vi "Additional Channels.vi"   [LabVIEW 2022 SP3]
uses:
  Controls/Post_Process.ctl
  Globals/Meas_global.vi
types:
  T1 = typedef "Analysis_info_cluster.ctl" = cluster{"Colour":u32, "Inst type":T2, "Inst name":string, "Symbol":string, "Code name":string, "Extra Info":string, "Inst Array":T3, "Extra Titles":string[], "Extra Values":string[], "U":dbl, "u^2":dbl, "u^3":dbl, "u^4":dbl, "Skew_u":dbl, "Kurt_u":dbl, "Sd Error in Mean":dbl, "% u'/U":dbl, "X":dbl, "Y":dbl, "Z":dbl, "Timescale integral Estimate":dbl, "Sd Error in Variance":dbl, "Calib File":path, "Calib Constants":dbl[], "Output Position":bool, "Stats":enum16{"None", "Basic", "Full"}, "Av Sampling Rate":dbl, "Av No of Samples":dbl, "Total Meas Time (s)":dbl, "ADAM Ch Name":string, "Max value":dbl, "Min value":dbl, "Req Sample Rate Hz":dbl, "Sync Delay Time (s)":dbl, "Ch No":i16, "Device":string, "Use Latest Calib":bool, "Port":string, "Metadata Ch Names":string[], "Metadata Ch Values":string[], "Label":string, "chState":T4}
  T2 = typedef "Inst_type.ctl" = enum16{"Raw voltage", "Raw with zero offsetting", "Propeller anemometer", "Pressure Transducer", "Pitot-static tube", "Hot wire", "Cross wire 1", "Cross wire 2", "Generic Linear", "Generic Polynomial", "Generic BackPoly", "Fast FID", "Thermocouple", "Cold wire", "Pulsed Wire", "LDA Vel", "LDA Tran time", "LDA Arr time", "Microphone"}
  T3 = typedef "Instrument_Array.ctl" = enum16{"PWA", "LDA", "Analogue"}
  T4 = typedef "channelState.ctl" = enum32{"No Selection", "Solo", "Mute"}
  T5 = typedef "Post_Process.ctl" = enum16{"Take New Data", "Post Process Raw Data File"}
  T6 = typedef "Initial Info Cluster.ctl" = cluster{"Metadata Ch Names":string[], "Metadata Ch Values":string[]}
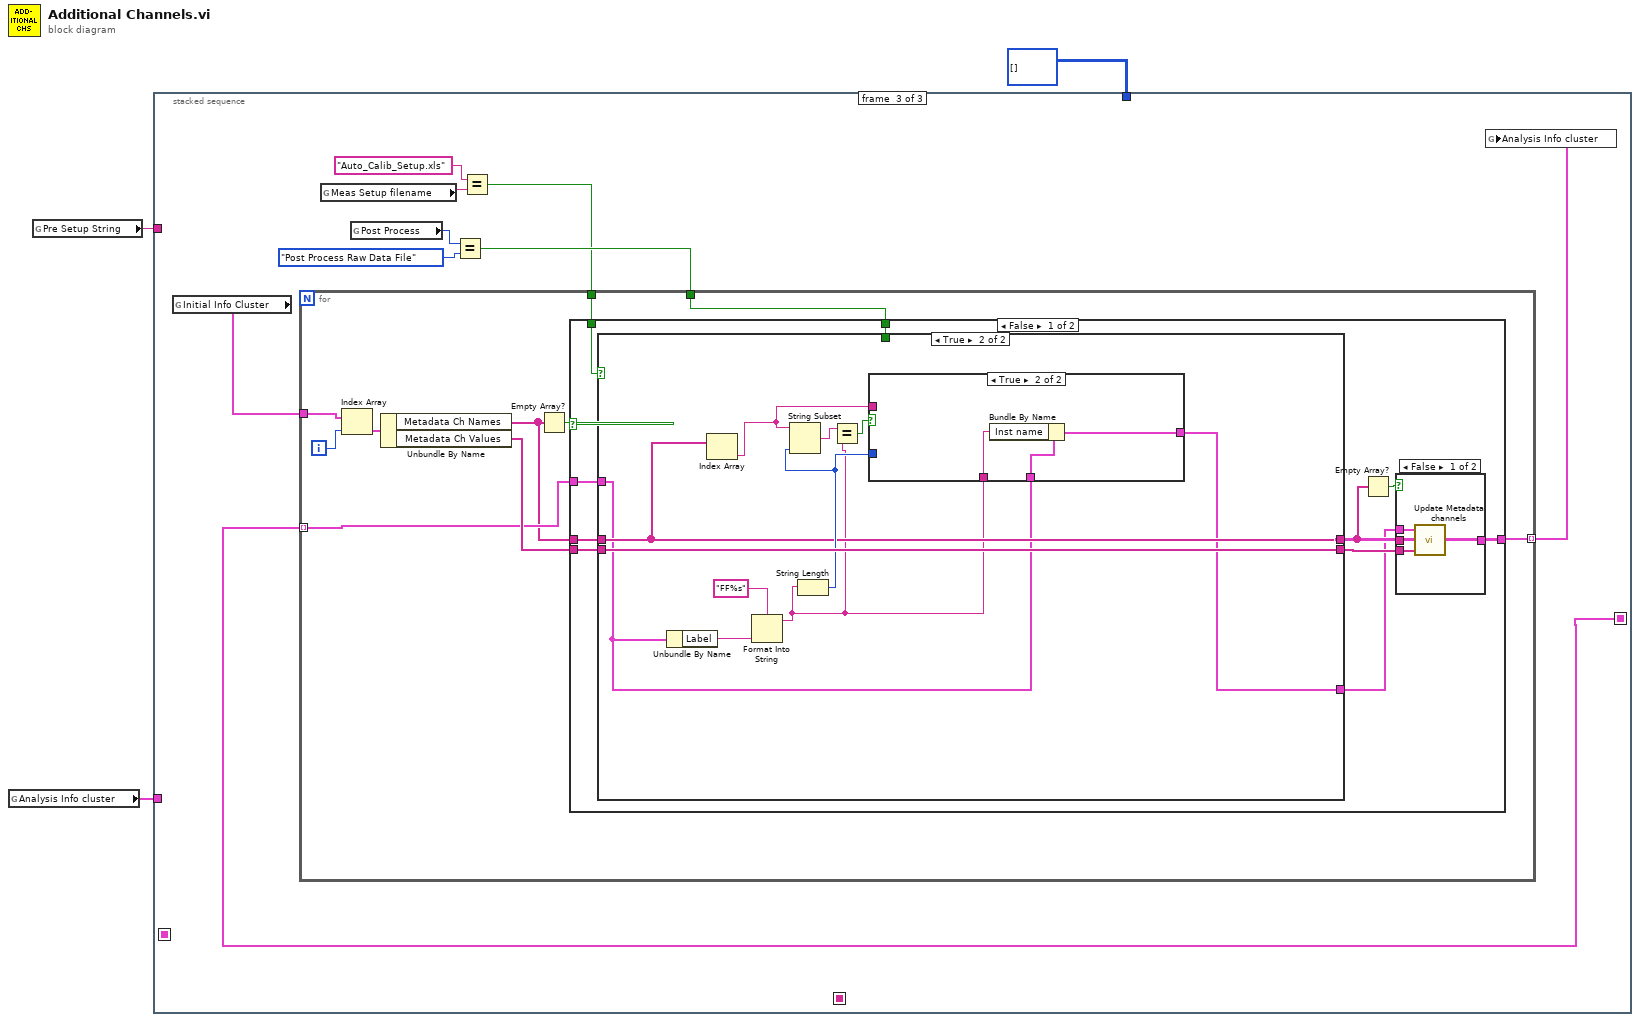
[diagram p0: block diagram]
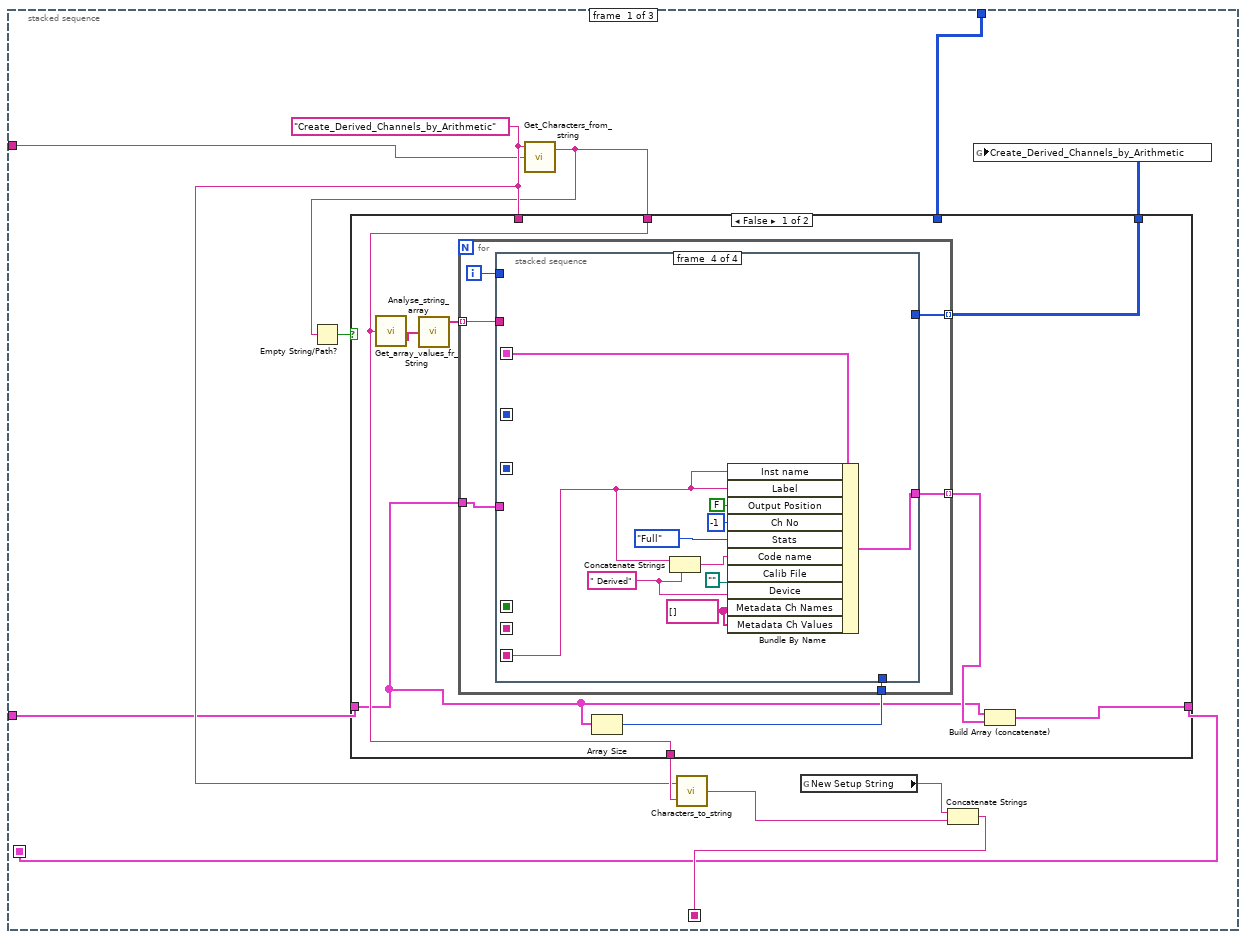
[diagram p2: hidden frame]
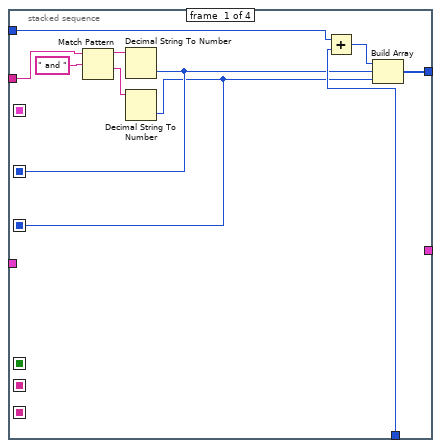
[diagram p3: hidden frame]
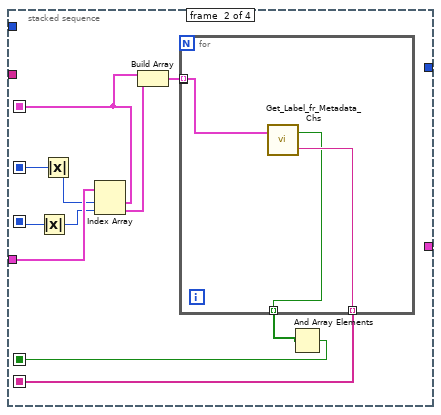
[diagram p4: hidden frame]
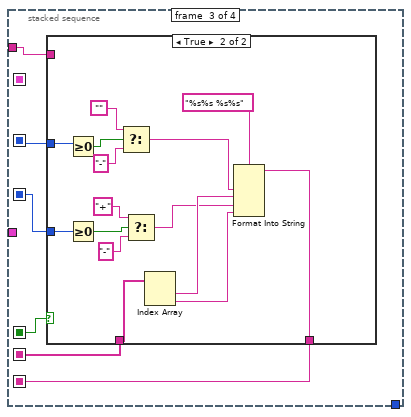
[diagram p5: hidden frame]
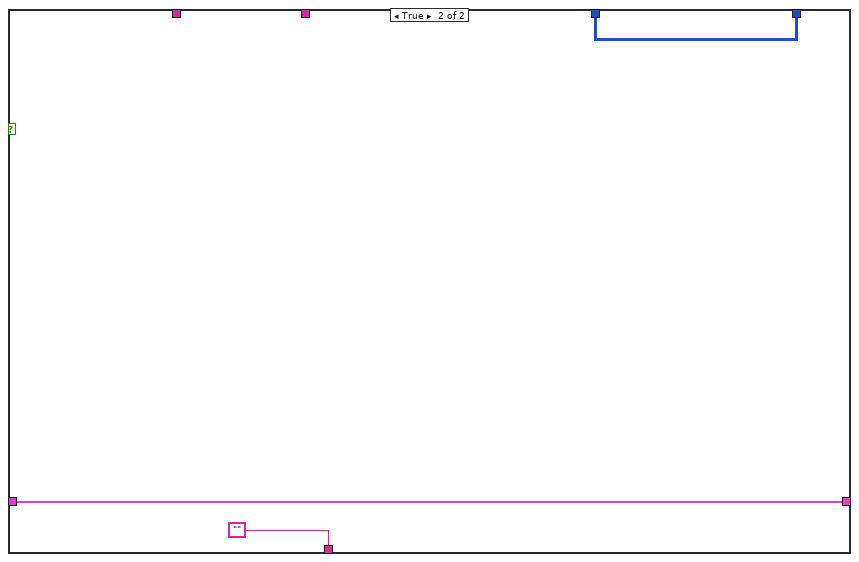
[diagram p7: hidden frame]
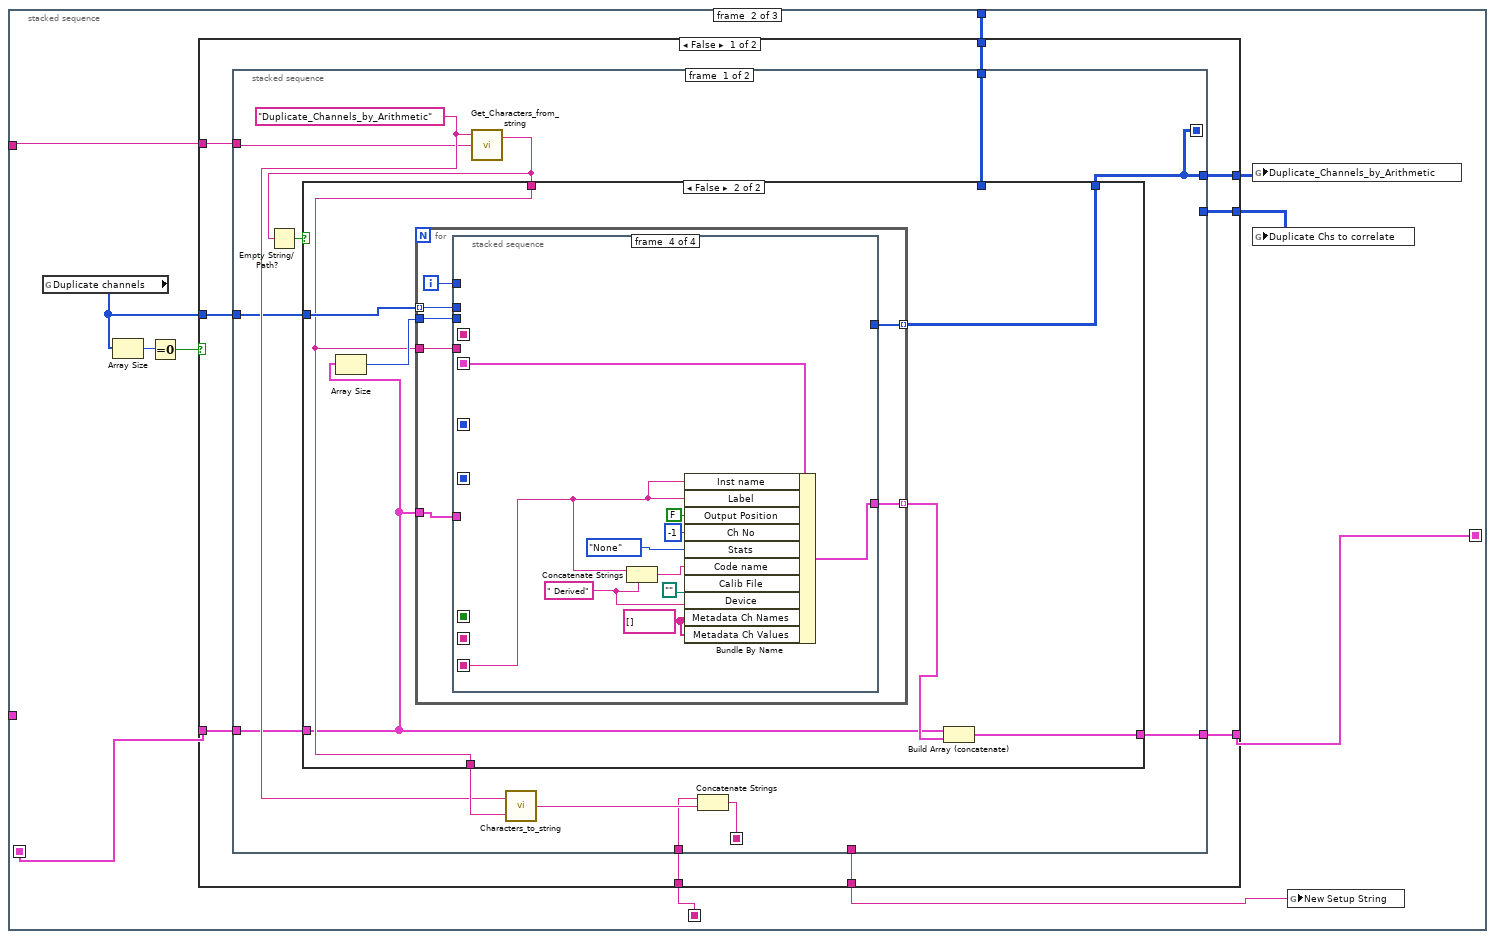
[diagram p8: hidden frame]
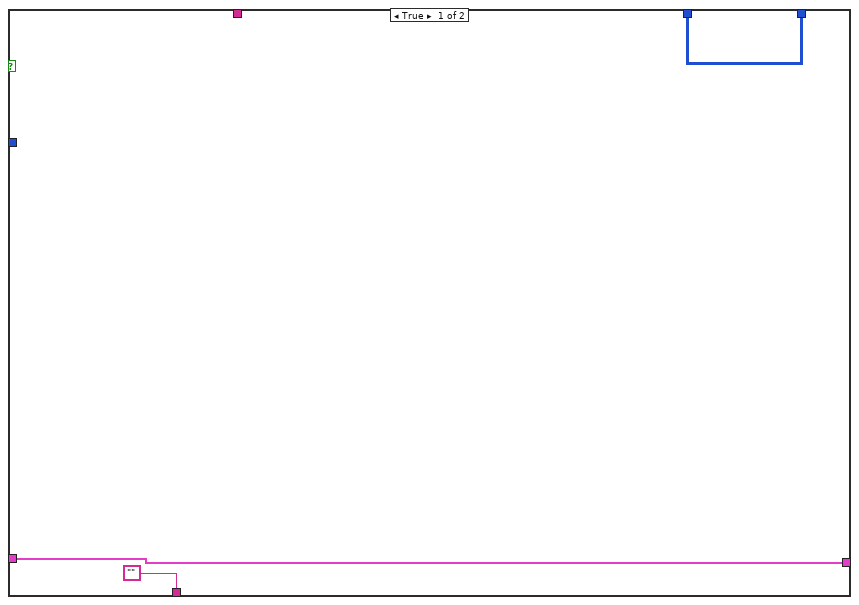
[diagram p9: hidden frame]
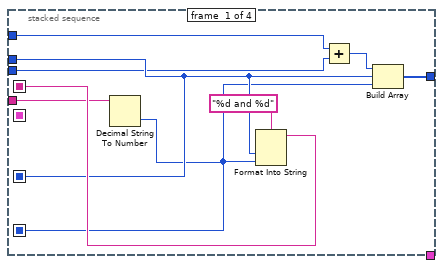
[diagram p10: hidden frame]
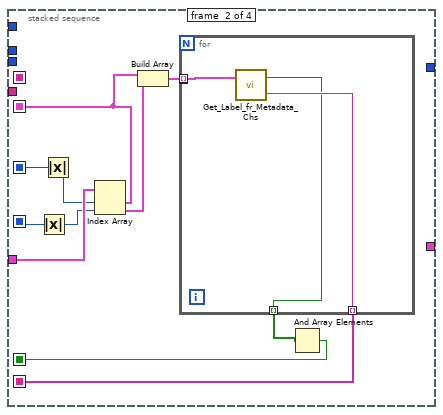
[diagram p11: hidden frame]
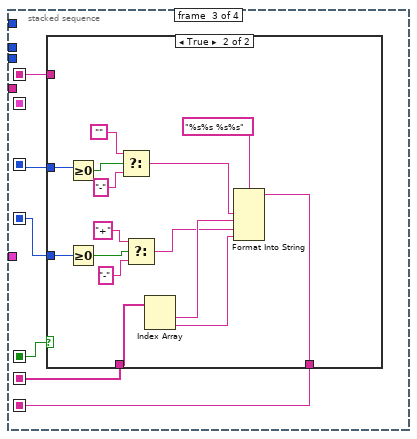
[diagram p12: hidden frame]
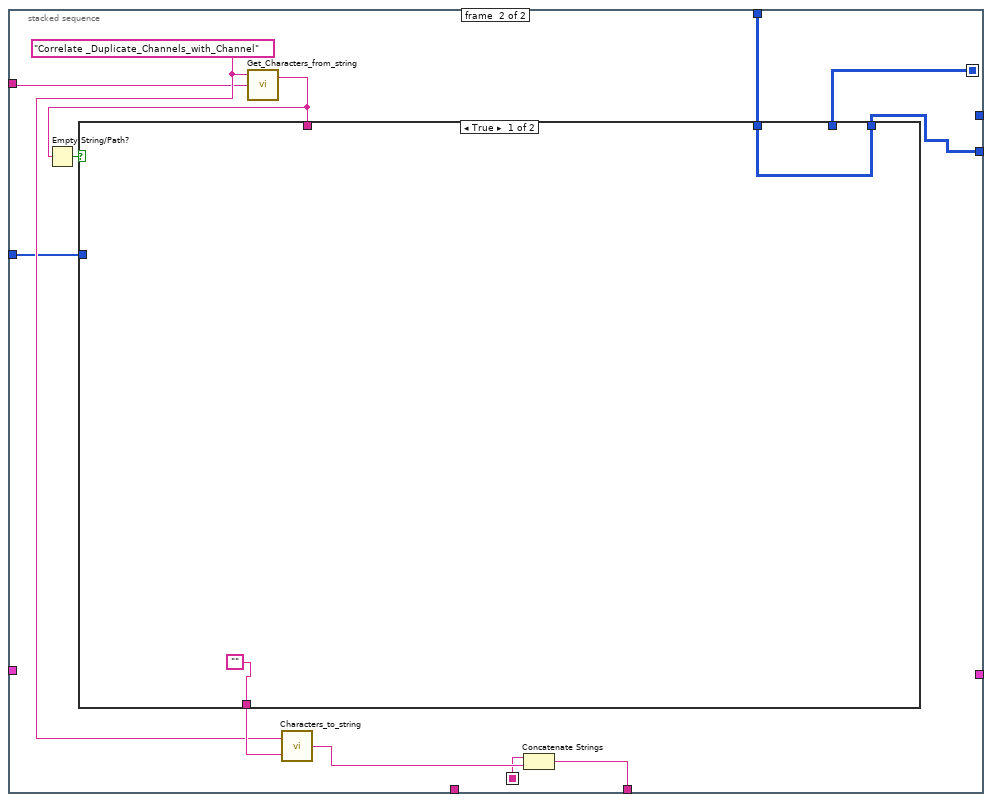
[diagram p14: hidden frame]
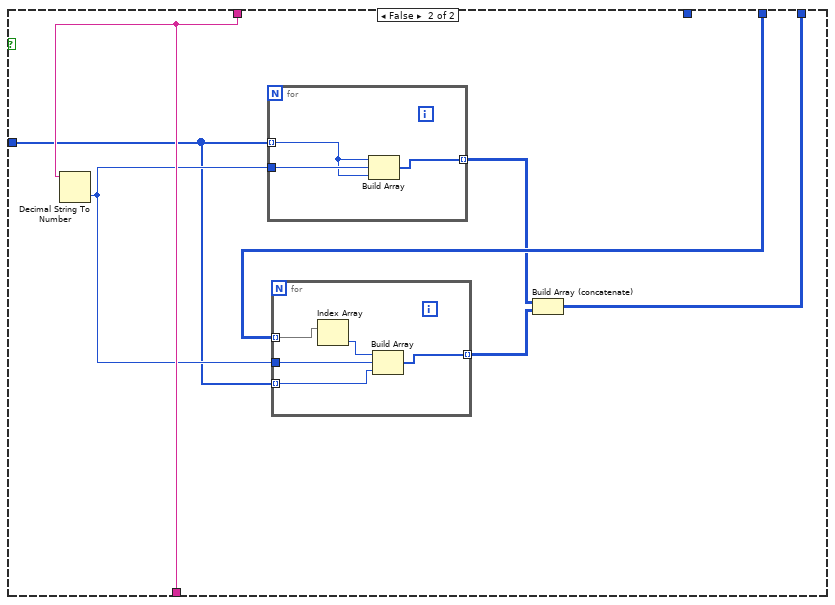
[diagram p15: hidden frame]
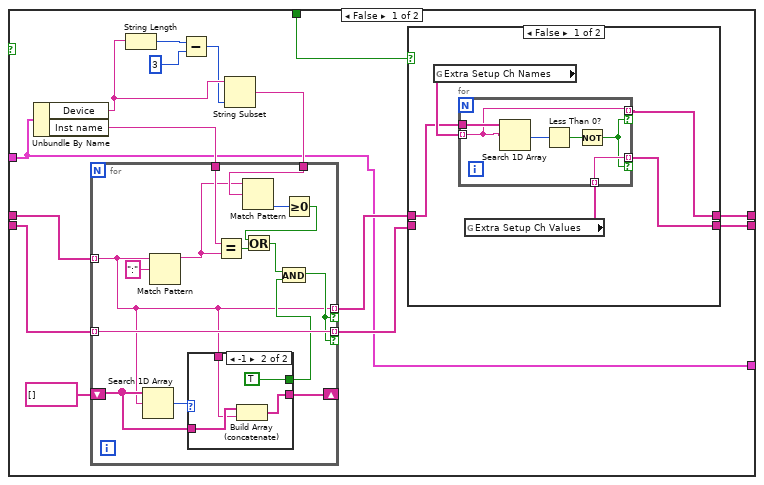
[diagram p17: hidden frame]
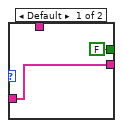
[diagram p18: hidden frame]
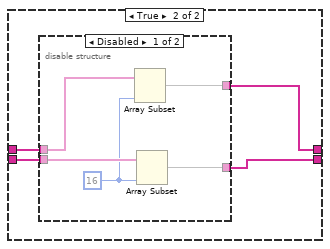
[diagram p19: hidden frame]
diagram:
  n1 = global read "Meas_global.vi" "Analysis Info cluster"() -> (w1:T1[])
  n2 = global read "Meas_global.vi" "Pre Setup String"() -> (w2:string)
  n3 = stacked-sequence {
    seq-local: [w10 _ _] -> [_ w92 _]
    seq-local: [w4 _ _] -> [_ w90 _]
    seq-local: [_ w89 _] -> [_ _ w233]
    tunnel: i32[][] [] -> [w8 w95 _]
    tunnel: w2 -> [w9 w94 _]
    tunnel: w1 -> [w5 _ _]
    frame #0 {
      w13 = "Create_Derived_Channels_by_Arithmetic"
      n4 = call "Get_Characters_from_string.vi"("Input string"=w9, "Variable name"=w13) -> ("Value"=w6:string)  [unwired: 1 in, 1 out]
      n5 = Empty String/Path?(string/path=w6) -> (empty?=w7:bool)
      n6 = case shown="False" w7 {
        tunnel: w6 -> [w18 _]
        tunnel: w13 -> [_ _]
        tunnel: [w20 w87] -> w11
        tunnel: [w18 ""] -> w15
        tunnel: w8 -> [_ w87]
        tunnel: w5 -> [w17 w86]
        tunnel: [w16 w86] -> w4
        frame False {
          n7 = call "Get_array_values_fr_String.vi"("String Value"=w18) -> ("String array"=w22:string[])  [unwired: 1 out]
          n8 = call "Analyse_string_array.vi"("String array"=w22) -> ("Unique strings"=w21:string[])  [unwired: 1 in, 1 out]
          n9 = Array Size(array=w17) -> (size(s)=w19:i32)
          n10 = for {
            tunnel: w21 -> [w28] mode=indexing
            tunnel: [w26] -> w20 mode=indexing
            tunnel: w17 -> [w29]
            tunnel: [w27] -> w23 mode=indexing
            tunnel: w19 -> [w24]
            i -> [w25]
            n11 = stacked-sequence {
              seq-local: [w31 _ _ _] -> [_ w49 w57 _]
              seq-local: [w30 _ _ _] -> [_ w48 w56 _]
              seq-local: [_ w45 _ _] -> [_ _ _ w77]
              seq-local: [_ w41 _ _] -> [_ _ w59 _]
              seq-local: [_ w40 _ _] -> [_ _ w58 _]
              seq-local: [_ _ w55 _] -> [_ _ _ w76]
              tunnel: w29 -> [_ w50 _ _]
              tunnel: w28 -> [w36 _ w54 _]
              tunnel: [_ _ _ w84] -> w27
              tunnel: [w35 _ _ _] -> w26
              tunnel: w25 -> [w34 _ _ _]
              tunnel: w24 -> [w32 _ _ _]
              frame #0 {
                n12 = Match Pattern(string=w36, regular expression=" and ") -> (before substring=w38:string, after substring=w37:string)  [unwired: 3 out]
                n13 = Decimal String To Number(string=w38) -> (number=w31:i32)  [unwired: 3 out]
                n14 = Decimal String To Number(string=w37) -> (number=w30:i32)  [unwired: 3 out]
                n15 = Add(x=w34, y=w32) -> (x+y=w33:i32)
                n16 = Build Array(w33, w31, w30) -> (w35:i32[])
              }
              frame #1 {
                n17 = Absolute Value(x=w48) -> (abs(x)=w46:i32)
                n18 = Absolute Value(x=w49) -> (abs(x)=w47:i32)
                n19 = Index Array(array=w50, index #1=w47, index #2=w46) -> (element #1=w45:T1, element #2=w44:T1)
                n20 = Build Array(w45, w44) -> (w43:T1[])
                n21 = for {
                  tunnel: [w53] -> _ mode=indexing
                  tunnel: w43 -> [w53] mode=indexing
                  tunnel: [w52] -> w40 mode=indexing
                  tunnel: [w51] -> w42 mode=indexing
                  n22 = call "Get_Label_fr_Metadata_Chs.vi"("Info Cluster"=w53) -> ("Label"=w52:string, "Label found?"=w51:bool)  [unwired: 1 in]
                }
                n23 = And Array Elements(Boolean array=w42) -> (logical AND=w41:bool)
              }
              frame #2 {
                n24 = case shown="True" w59 {
                  tunnel: w58 -> [_ w75]
                  tunnel: w57 -> [_ w62]
                  tunnel: w56 -> [_ w69]
                  tunnel: [w60 w63] -> w55
                  tunnel: w54 -> [w60 _]
                  frame False {
                  }
                  frame True {
                    n25 = Greater Or Equal To 0?(x=w62) -> (x >= 0?=w61:bool)
                    n26 = Greater Or Equal To 0?(x=w69) -> (x >= 0?=w70:bool)
                    n27 = Select(t="", s=w61, f="-") -> (s? t:f=w68:string)
                    n28 = Select(t="+", s=w70, f="-") -> (s? t:f=w66:string)
                    n29 = Index Array(array=w75) -> (element #1=w67:string, element #2=w65:string)  [unwired: 2 in]
                    n30 = Format Into String(format string="%s%s %s%s", w68, w67, w66, w65) -> (resulting string=w63:string)  [unwired: 2 in, 1 out]
                  }
                }
              }
              frame #3 {
                w79 = string[] [] ("Metadata Ch Names")
                w85 = " Derived"
                n31 = Concatenate Strings(w76, w85) -> (w81:string)
                n32 = Bundle By Name(cluster=w77, "Inst name"=w76, "Label"=w76, "Output Position"=FALSE, "Ch No"=i16 -1, "Stats"=enum16{"None", "Basic", "Full"}."Full", "Code name"=w81, "Calib File"=path "", "Device"=w85, "Metadata Ch Names"=w79, "Metadata Ch Values"=w79) -> (w84:T1)
              }
            }
          }
          n33 = Build Array (concatenate)(w17, w23) -> (w16:T1[])
        }
        frame True {
        }
      }
      n34 = call "Characters_to_string.vi"("Characters to write"=w15, "Label for characters"=w13) -> ("Output string"=w14:string)  [unwired: 1 in]
      n35 = global read "Meas_global.vi" "New Setup String"() -> (w12:string)
      n36 = Concatenate Strings(w12, w14) -> (w10:string)
      n37 = global write "Meas_global.vi" "Create_Derived_Channels_by_Arithmetic"(w11) -> ()
    }
    frame #1 {
      n38 = global read "Meas_global.vi" "Duplicate channels"() -> (w99:i32[])
      n39 = Array Size(array=w99) -> (size(s)=w98:i32)
      n40 = Equal To 0?(x=w98) -> (x = 0?=w97:bool)
      n41 = case shown="False" w97 {
        tunnel: w99 -> [w108 _]
        tunnel: [w106 w225] -> w96
        tunnel: w95 -> [w107 w225]
        tunnel: w94 -> [w105 _]
        tunnel: [w104 w225] -> w93
        tunnel: w92 -> [w103 w224]
        tunnel: [w102 w224] -> w91
        tunnel: w90 -> [w101 w223]
        tunnel: [w100 w223] -> w89
        frame False {
          n42 = stacked-sequence {
            seq-local: [w114 _] -> [_ w198]
            seq-local: [w113 _] -> [_ w196]
            tunnel: w108 -> [w118 w202]
            tunnel: w107 -> [w117 w201]
            tunnel: [w113 _] -> w106
            tunnel: w105 -> [w116 w200]
            tunnel: w103 -> [w115 _]
            tunnel: [_ w199] -> w102
            tunnel: [_ w197] -> w104
            tunnel: w101 -> [w110 _]
            tunnel: [w109 _] -> w100
            frame #0 {
              w120 = "Duplicate_Channels_by_Arithmetic"
              n43 = call "Get_Characters_from_string.vi"("Input string"=w116, "Variable name"=w120) -> ("Value"=w112:string)  [unwired: 1 in, 1 out]
              n44 = Empty String/Path?(string/path=w112) -> (empty?=w111:bool)
              n45 = case shown="False" w111 {
                tunnel: [w123 w130] -> w113
                tunnel: ["" w127] -> w121
                tunnel: w112 -> [_ w127]
                tunnel: w118 -> [_ w128]
                tunnel: w117 -> [w123 _]
                tunnel: w110 -> [w122 w126]
                tunnel: [w122 w125] -> w109
                frame True {
                }
                frame False {
                  n46 = Array Size(array=w126) -> (size(s)=w129:i32)
                  n47 = for {
                    tunnel: [w136] -> w130 mode=indexing
                    tunnel: w126 -> [w138]
                    tunnel: [w137] -> w131 mode=indexing
                    tunnel: w128 -> [w134] mode=indexing
                    tunnel: w129 -> [w133]
                    tunnel: w127 -> [w132]
                    i -> [w135]
                    n48 = stacked-sequence {
                      seq-local: [w144 _ _ _] -> [_ w157 w165 _]
                      seq-local: [w139 _ _ _] -> [_ w156 w164 _]
                      seq-local: [_ w155 _ _] -> [_ _ _ w185]
                      seq-local: [_ w151 _ _] -> [_ _ w167 _]
                      seq-local: [_ w150 _ _] -> [_ _ w166 _]
                      seq-local: [_ _ w163 _] -> [_ _ _ w184]
                      seq-local: [w145 _ _ _] -> [_ _ w162 _]
                      tunnel: w138 -> [_ w158 _ _]
                      tunnel: [_ _ _ w192] -> w137
                      tunnel: [w147 _ _ _] -> w136
                      tunnel: w135 -> [w143 _ _ _]
                      tunnel: w134 -> [w144 _ _ _]
                      tunnel: w133 -> [w141 _ _ _]
                      tunnel: w132 -> [w140 _ _ _]
                      frame #0 {
                        n49 = Decimal String To Number(string=w140) -> (number=w139:i32)  [unwired: 2 in, 1 out]
                        n50 = Format Into String(format string="%d and %d", w144, w139) -> (resulting string=w145:string)  [unwired: 2 in, 1 out]
                        n51 = Add(x=w143, y=w141) -> (x+y=w142:i32)
                        n52 = Build Array(w142, w144, w139) -> (w147:i32[])
                      }
                      frame #1 {
                        n53 = Absolute Value(x=w156) -> (abs(x)=w148:i32)
                        n54 = Absolute Value(x=w157) -> (abs(x)=w149:i32)
                        n55 = Index Array(array=w158, index #1=w149, index #2=w148) -> (element #1=w155:T1, element #2=w154:T1)
                        n56 = Build Array(w155, w154) -> (w153:T1[])
                        n57 = for {
                          tunnel: [w161] -> _ mode=indexing
                          tunnel: w153 -> [w161] mode=indexing
                          tunnel: [w160] -> w150 mode=indexing
                          tunnel: [w159] -> w152 mode=indexing
                          n58 = call "Get_Label_fr_Metadata_Chs.vi"("Info Cluster"=w161) -> ("Label"=w160:string, "Label found?"=w159:bool)  [unwired: 1 in]
                        }
                        n59 = And Array Elements(Boolean array=w152) -> (logical AND=w151:bool)
                      }
                      frame #2 {
                        n60 = case shown="True" w167 {
                          tunnel: w166 -> [_ w183]
                          tunnel: w165 -> [_ w170]
                          tunnel: w164 -> [_ w177]
                          tunnel: [w168 w171] -> w163
                          tunnel: w162 -> [w168 _]
                          frame False {
                          }
                          frame True {
                            n61 = Greater Or Equal To 0?(x=w170) -> (x >= 0?=w169:bool)
                            n62 = Greater Or Equal To 0?(x=w177) -> (x >= 0?=w178:bool)
                            n63 = Select(t="", s=w169, f="-") -> (s? t:f=w176:string)
                            n64 = Select(t="+", s=w178, f="-") -> (s? t:f=w174:string)
                            n65 = Index Array(array=w183) -> (element #1=w175:string, element #2=w173:string)  [unwired: 2 in]
                            n66 = Format Into String(format string="%s%s %s%s", w176, w175, w174, w173) -> (resulting string=w171:string)  [unwired: 2 in, 1 out]
                          }
                        }
                      }
                      frame #3 {
                        w187 = string[] [] ("Metadata Ch Names")
                        w193 = " Derived"
                        n67 = Concatenate Strings(w184, w193) -> (w189:string)
                        n68 = Bundle By Name(cluster=w185, "Inst name"=w184, "Label"=w184, "Output Position"=FALSE, "Ch No"=i16 -1, "Stats"=enum16{"None", "Basic", "Full"}."None", "Code name"=w189, "Calib File"=path "", "Device"=w193, "Metadata Ch Names"=w187, "Metadata Ch Values"=w187) -> (w192:T1)
                      }
                    }
                  }
                  n69 = Build Array (concatenate)(w126, w131) -> (w125:T1[])
                }
              }
              n70 = call "Characters_to_string.vi"("Characters to write"=w121, "Label for characters"=w120) -> ("Output string"=w119:string)  [unwired: 1 in]
              n71 = Concatenate Strings(w115, w119) -> (w114:string)
            }
            frame #1 {
              w204 = "Correlate _Duplicate_Channels_with_Channel"
              n72 = call "Get_Characters_from_string.vi"("Input string"=w200, "Variable name"=w204) -> ("Value"=w194:string)  [unwired: 1 in, 1 out]
              n73 = Empty String/Path?(string/path=w194) -> (empty?=w195:bool)
              n74 = case shown="True" w195 {
                tunnel: [w206 w209] -> w197
                tunnel: ["" w214] -> w205
                tunnel: w194 -> [_ w214]
                tunnel: w202 -> [_ w208]
                tunnel: w201 -> [w206 _]
                tunnel: w196 -> [_ w212]
                frame True {
                }
                frame False {
                  n75 = Decimal String To Number(string=w214) -> (number=w213:i32)  [unwired: 2 in, 1 out]
                  n76 = for {
                    tunnel: [w222] -> w210 mode=indexing
                    tunnel: w208 -> [w220] mode=indexing
                    tunnel: w213 -> [w221]
                    n77 = Build Array(w220, w221, w220) -> (w222:i32[])
                  }
                  n78 = for {
                    tunnel: [w219] -> w211 mode=indexing
                    tunnel: w212 -> [w217] mode=indexing
                    tunnel: w213 -> [w218]
                    tunnel: w208 -> [w215] mode=indexing
                    n79 = Index Array(array=w217) -> (element=w216:i32)  [unwired: 1 in]
                    n80 = Build Array(w216, w218, w215) -> (w219:i32[])
                  }
                  n81 = Build Array (concatenate)(w210, w211) -> (w209:i32[][])
                }
              }
              n82 = call "Characters_to_string.vi"("Characters to write"=w205, "Label for characters"=w204) -> ("Output string"=w203:string)  [unwired: 1 in]
              n83 = Concatenate Strings(w198, w203) -> (w199:string)
            }
          }
        }
        frame True {
        }
      }
      n84 = global write "Meas_global.vi" "Duplicate_Channels_by_Arithmetic"(w96) -> ()
      n85 = global write "Meas_global.vi" "Duplicate Chs to correlate"(w93) -> ()
      n86 = global write "Meas_global.vi" "New Setup String"(w91) -> ()
    }
    frame #2 {
      n87 = global read "Meas_global.vi" "Initial Info Cluster"() -> (w234:T6[])
      n88 = global read "Meas_global.vi" "Meas Setup filename"() -> (w228:string)
      n89 = global read "Meas_global.vi" "Post Process"() -> (w230:T5)
      n90 = Equal?(x=w230, y=Post_Process."Post Process Raw Data File" ("Post Process")) -> (x = y?=w229:bool)
      n91 = Equal?(x="Auto_Calib_Setup.xls", y=w228) -> (x = y?=w226:bool)
      n92 = for {
        tunnel: w234 -> [w242]
        tunnel: w233 -> [w237] mode=indexing
        tunnel: [w243] -> w232 mode=indexing
        tunnel: w229 -> [w239]
        tunnel: w226 -> [w236]
        i -> [w241]
        n93 = Index Array(array=w242, index=w241) -> (element=w240:T6)
        n94 = Unbundle By Name(w240) -> ("Metadata Ch Names"=w235:string[], "Metadata Ch Values"=w244:string[])
        n95 = Empty Array?(array=w235) -> (empty?=w238:bool)
        n96 = case shown="False" w238 {
          tunnel: w237 -> [w246 w333]
          tunnel: w235 -> [w249 _]
          tunnel: w244 -> [w248 _]
          tunnel: [w254 w333] -> w243
          tunnel: w239 -> [w250 _]
          tunnel: w236 -> [w247 _]
          frame False {
            n97 = case shown="True" w247 {
              tunnel: [w269 w323] -> w253
              tunnel: [w268 w316] -> w252
              tunnel: w250 -> [w267 _]
              tunnel: w246 -> [w255 w315]
              tunnel: w249 -> [w266 w316]
              tunnel: w248 -> [w262 w323]
              tunnel: [w255 w313] -> w245
              frame False {
                n98 = Unbundle By Name(w255) -> ("Device"=w258:string, "Inst name"=w265:string)
                n99 = String Length(string=w258) -> (length=w260:i32)
                n100 = Subtract(x=w260, y=3) -> (x-y=w257:i32)
                n101 = String Subset(string=w258, length (rest)=w257) -> (substring=w256:string)  [unwired: 1 in]
                n102 = for {
                  tunnel: w266 -> [w276] mode=indexing
                  tunnel: w265 -> [w283]
                  tunnel: [w276] -> w264 mode=indexing if=w277
                  tunnel: [w282] -> w263 mode=indexing if=w277
                  tunnel: w262 -> [w282] mode=indexing
                  shift-right: [w279] -> _
                  shift-left: string[] [] -> [w280]
                  tunnel: w256 -> [w275]
                  n103 = Search 1D Array(1D array=w280, element=w276) -> (index of element=w281:i32)  [unwired: 1 in]
                  n104 = Match Pattern(string=w276, regular expression=":") -> (before substring=w274:string)  [unwired: 1 in, 3 out]
                  n105 = case shown="-1" w281 {
                    tunnel: w280 -> [w286 w290]
                    tunnel: w276 -> [_ w289]
                    tunnel: [w286 w288] -> w279
                    tunnel: [FALSE TRUE] -> w278
                    frame Default {
                    }
                    frame -1 {
                      n106 = Build Array (concatenate)(w290, w289) -> (w288:string[])
                    }
                  }
                  n107 = Equal?(x=w283, y=w274) -> (x = y?=w271:bool)
                  n108 = Match Pattern(string=w274, regular expression=w275) -> (offset past match=w273:i32)  [unwired: 1 in, 3 out]
                  n109 = Greater Or Equal To 0?(x=w273) -> (x >= 0?=w272:bool)
                  n110 = Or(x=w272, y=w271) -> (x .or. y?=w270:bool)
                  n111 = And(x=w270, y=w278) -> (x .and. y?=w277:bool)
                }
                n112 = case shown="False" w267 {
                  tunnel: w264 -> [w294 w305]
                  tunnel: [w293 w303] -> w269
                  tunnel: [w291 w302] -> w268
                  tunnel: w263 -> [_ w304]
                  frame False {
                    n113 = global read "Meas_global.vi" "Extra Setup Ch Names"() -> (w295:string[])
                    n114 = global read "Meas_global.vi" "Extra Setup Ch Values"() -> (w292:string[])
                    n115 = for {
                      tunnel: w294 -> [w301]
                      tunnel: w295 -> [w298] mode=indexing
                      tunnel: [w298] -> w291 mode=indexing if=w296
                      tunnel: [w297] -> w293 mode=indexing if=w296
                      tunnel: w292 -> [w297] mode=indexing
                      n116 = Search 1D Array(1D array=w301, element=w298) -> (index of element=w300:i32)  [unwired: 1 in]
                      n117 = Less Than 0?(x=w300) -> (x < 0?=w299:bool)
                      n118 = Not(x=w299) -> (.not. x?=w296:bool)
                    }
                  }
                  frame True {
                    n119 = disable-structure shown="Disabled" {
                      disable-tunnel: w305 -> [w310 w312]
                      disable-tunnel: w304 -> [w309 w311]
                      disable-tunnel: [w308 w311] -> w303
                      disable-tunnel: [w307 w312] -> w302
                      frame Disabled {
                        w306 = 16 ("length")
                        n120 = Array Subset(array=w310, length=w306) -> (w307:string[])  [unwired: 1 in]
                        n121 = Array Subset(array=w309, length=w306) -> (w308:string[])  [unwired: 1 in]
                      }
                      frame Enabled {
                      }
                    }
                  }
                }
              }
              frame True {
                n122 = Unbundle By Name(w315) -> ("Label"=w321:string)
                n123 = Index Array(array=w316) -> (element=w317:string)  [unwired: 1 in]
                n124 = Format Into String(format string="FF%s", w321) -> (resulting string=w314:string)  [unwired: 2 in, 1 out]
                n125 = String Length(string=w314) -> (length=w320:i32)
                n126 = String Subset(string=w317, length (rest)=w320) -> (substring=w319:string)  [unwired: 1 in]
                n127 = Equal?(x=w319, y=w314) -> (x = y?=w318:bool)
                n128 = case shown="True" w318 {
                  tunnel: w320 -> [_ _]
                  tunnel: w317 -> [_ _]
                  tunnel: w315 -> [w324 w327]
                  tunnel: w314 -> [_ w326]
                  tunnel: [w324 w325] -> w313
                  frame False {
                  }
                  frame True {
                    n129 = Bundle By Name(cluster=w327, "Inst name"=w326) -> (w325:T1)
                  }
                }
              }
            }
            n130 = Empty Array?(array=w252) -> (empty?=w251:bool)
            n131 = case shown="False" w251 {
              tunnel: w245 -> [w331 w332]
              tunnel: w252 -> [w330 _]
              tunnel: w253 -> [w329 _]
              tunnel: [w328 w332] -> w254
              frame False {
                n132 = call "Update Metadata channels.vi"("Metadata Values"=w329, "Metadata Names"=w330, "Analysis info Cluster in"=w331) -> ("Analysis info Cluster out"=w328:T1)
              }
              frame True {
              }
            }
          }
          frame True {
          }
        }
      }
      n133 = global write "Meas_global.vi" "Analysis Info cluster"(w232) -> ()
    }
  }
